vi "ATMonochromator_issueCommand_changeSlitWidth.vi"(8 "error in (no error)":errorcluster, 11 "command_changeSlitWidth_Ctl":T1) -> (0 "error out":errorcluster, 2 "function return":i32, 3 "command_changeSlitWidth_Ctl out":T1)   [LabVIEW 2016, in "SALLV_ATMonochromator.lvlib"]
doc: "int ATMonochromator_shm_issueCommand_changeSlitWidthLV(ATMonochromator_command_changeSlitWidthLV *command_changeSlitWidth_Ctl );"
uses:
  SALLV_ATMonochromator.lvlib
  DataTypes/command_changeSlitWidth.ctl
  SALLV_ATMonochromator.so
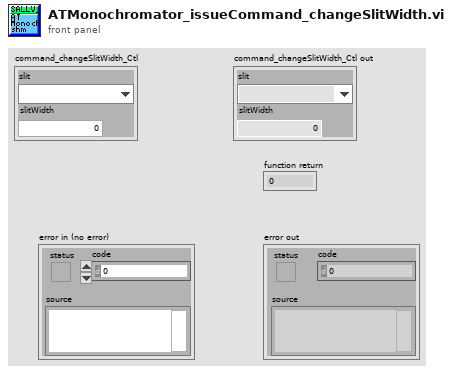
[diagram p1: front panel]
types:
  T1 = typedef "SALLV_ATMonochromator.lvlib/command_changeSlitWidth.ctl" = cluster{"slit":enum32{"", "FrontEntrance", "FrontExit"}, "slitWidth":sgl}
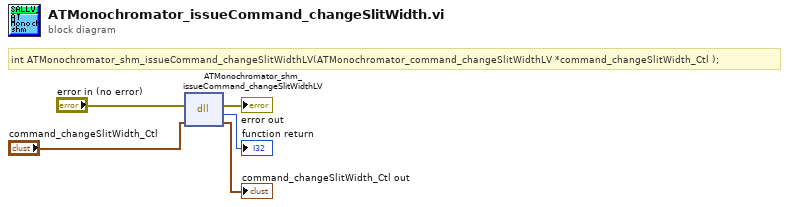
[diagram p0: block diagram]
diagram:
  # "int ATMonochromator_shm_issueCommand_changeSlitWidthLV(ATMonochromator_command_changeSlitWidthLV *command_changeSlitWidth_Ctl );"
  n1 = dll-call lib="home/harini/tcs/SALLV_ATMonochromator/SALLV_ATMonochromator.*" fn="ATMonochromator_shm_issueCommand_changeSlitWidthLV"(error in="error in (no error)", "command_changeSlitWidth_Ctl"="command_changeSlitWidth_Ctl") -> (error out=→"error out":errorcluster, →"function return":i32, "command_changeSlitWidth_Ctl"=→"command_changeSlitWidth_Ctl out":T1)  [unwired: 2 in, 1 out]
